vi "Find Mic Snippet.vi"() -> (0 "Mic B Device":dbl, 1 "Mic A Device":dbl, 2 "Number of Output Devices":i32, 3 "Number of Input Devices":i32, 4 "Speaker Device":dbl, 5 "Compensation factor":dbl, 6 "Faulty Mic":bool, 10 "Speaker Not Found":bool=TRUE)   [LabVIEW 2018]
uses:
  <vilib>/sound2/lvsound2.llb/Sound Data Format.ctl
  <vilib>/sound2/lvsound2.llb/Sampling Mode.ctl
  <vilib>/sound2/lvsound2.llb/Sound Output Set Volume (Single).vi
  <vilib>/sound2/lvsound2.llb/Sound Output Write (DBL Single).vi
  <vilib>/sound2/lvsound2.llb/Sound Input Read (DBL).vi
  <vilib>/addons/Sound and Vibration/svt_Level/SVT Sound Level (N Ch).vi
  <vilib>/measure/NI_MABase.lvlib
  <vilib>/addons/Sound and Vibration/svt_Level/SoundVib_SoundLevel.lvlib
panel:
  out "Filtered Signal 2":dynamicdata(graph) caption="Filtered Signal"
  out "Filtered Signal":dynamicdata(graph)
  out "db B":dbl
  out "db A":dbl
  out "Speaker Device 2":dbl
  out "equalized":dbl
  out "db Difference":dbl
  out "mv 2":dbl
  out "mv":dbl
  out "Number of Input Devices 2":i32
  in  "Boolean":bool
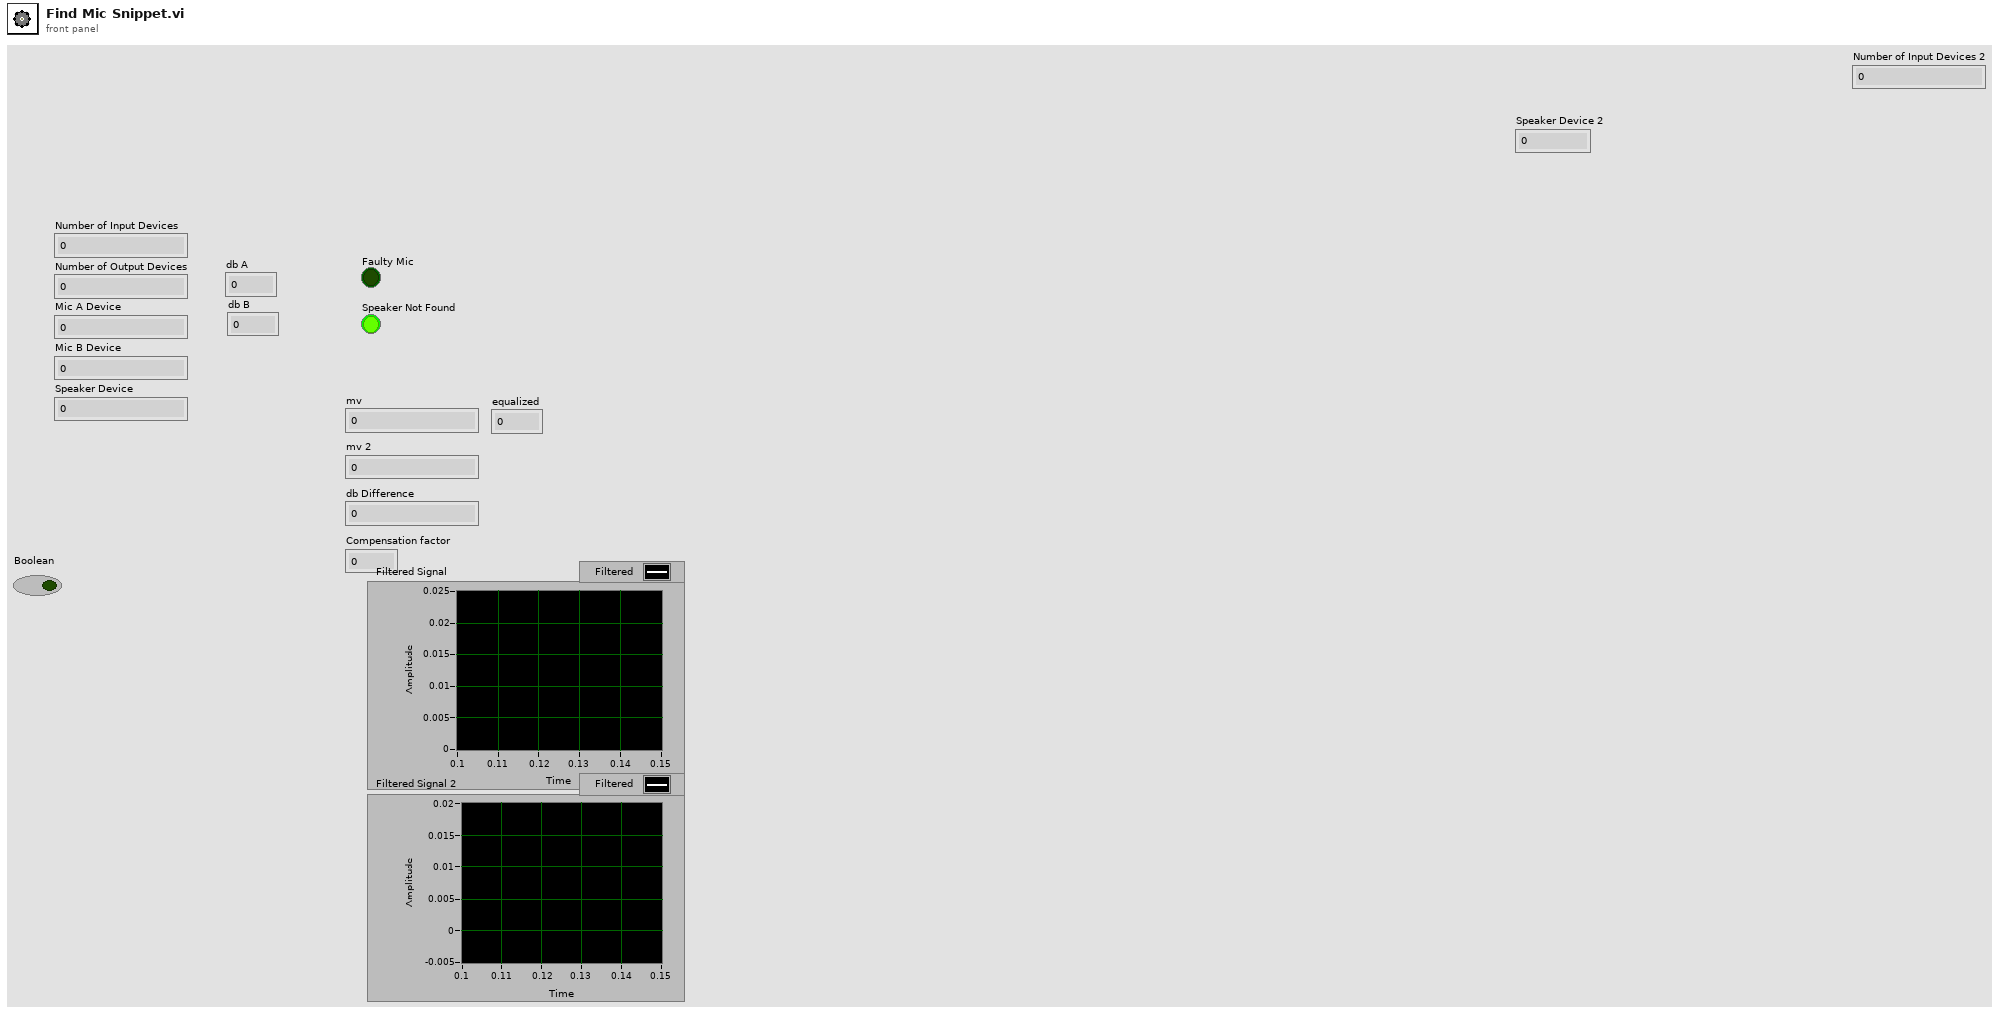
[diagram p1: front panel]
types:
  T1 = typedef "Sound Data Format.ctl" = cluster{"sample rate (S/s)":dbl, "number of channels":i32, "bits per sample":i32}
  T2 = cluster{"Leq":bool, "Running Leq":bool, "Exponential":bool, "Peak":bool}
  T3 = typedef "Sampling Mode.ctl" = i32
  T4 = typedef "Sound Output Task ID.ctl" = u32
  T5 = typedef "Sound Input Task ID.ctl" = u32
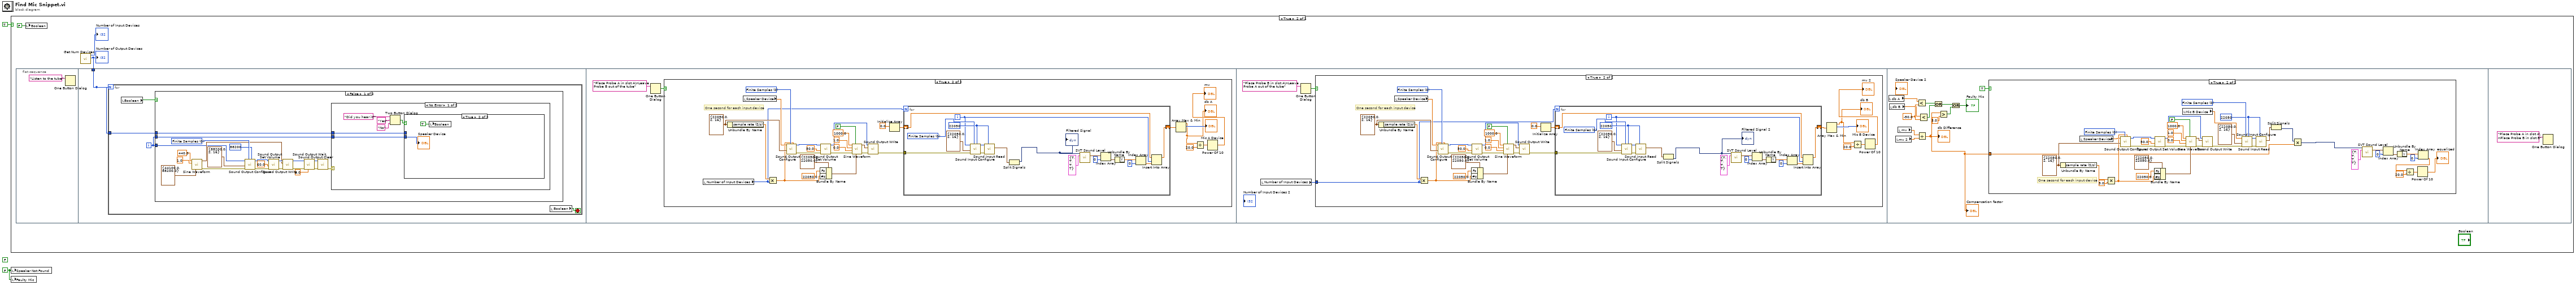
[diagram p0: block diagram]
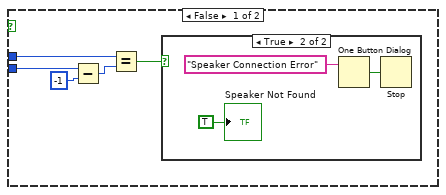
[diagram p3: hidden frame]
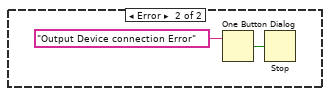
[diagram p5: hidden frame]
diagram:
  (unwired) FALSE
  w2 = FALSE
  n1 = case shown="True" TRUE {
    frame False {
    }
    frame True {
      n2 = flat-sequence {
        tunnel: w4 -> [w7]
        frame #0 {
          n3 = One Button Dialog(message="Listen to the tube") -> ()  [unwired: 1 in, 1 out]
        }
        frame #1 {
          n4 = for {
            N: w7 -> [_]
            tunnel: w7 -> [w8]
            i -> [w9]
            stop <- w11 stop-if-true
            n5 = local read "Boolean"() -> (w10:bool)
            n6 = case shown="False" w10 {
              tunnel: w9 -> [w14 _]
              tunnel: w9 -> [w13 _]
              tunnel: w8 -> [w12 _]
              frame False {
                w28 = T3 0 items=["Finite Samples", "Continuous Samples"] ("sample mode")
                n7 = call <vilib>:"Sine Waveform.vi"("sampling info"=cluster{"Fs":dbl, "#s":dbl} {"Fs"=44100.0, "#s"=88200.0}, "amplitude"=1.0, "frequency"=440.0) -> ("error out"=w31:errorcluster, "signal out"=w21:waveform(dbl))  [unwired: 7 in]
                n8 = call <vilib>:"Sound Output Configure.vi"("number of samples/ch"=88200, "sample mode"=w28, "error in (no error)"=w31, "sound format"=T1 {"sample rate (S/s)"=88200.0, "number of channels"=2, "bits per sample"=16}, "device ID"=w13) -> ("error out"=w26:errorcluster, "task ID"=w25:T4)  [unwired: 5 in]
                n9 = call-poly <vilib>:"Sound Output Set Volume.vi"("error in (no error)"=w26, "volume"=60.0, "task ID"=w25) -> ("error out"=w23:errorcluster, "task ID out"=w22:T4)  [unwired: 7 in]
                n10 = call-poly <vilib>:"Sound Output Write.vi"("error in (no error)"=w23, "data"=w21, "task ID"=w22) -> ("error out"=w20:errorcluster, "task ID out"=w19:T4)  [unwired: 7 in]
                n11 = call <vilib>:"Sound Output Wait.vi"("timeout (sec)"=2.0, "error in (no error)"=w20, "task ID"=w19) -> ("error out"=w17:errorcluster, "task ID out"=w16:T4)  [unwired: 7 in]
                n12 = call <vilib>:"Sound Output Clear.vi"("error in (no error)"=w17, "task ID"=w16) -> ("error out"=w15:errorcluster)  [unwired: 9 in]
                n13 = case shown="No Error" w15 {
                  tunnel: w14 -> [w35 _]
                  tunnel: w12 -> [w34 _]
                  frame No Error {
                    n14 = Two Button Dialog(message="Did you hear it?", 1:"No" ("F button name (\"Cancel\")"), 2:"Yes" ("T button name (\"OK\")")) -> (T button?=w36:bool)
                    n15 = case shown="True" w36 {
                      tunnel: w35 -> [w42 w48]
                      tunnel: w34 -> [w43 _]
                      frame False {
                        n16 = Subtract(x=w42, y=-1) -> (x-y=w40:i32)
                        n17 = Equal?(x=w43, y=w40) -> (x = y?=w44:bool)
                        n18 = case shown="True" w44 {
                          frame False {
                          }
                          frame True {
                            n19 = One Button Dialog(message="Speaker Connection Error") -> (true=w46:bool)  [unwired: 1 in]
                            n20 = Stop(stop? (T)=w46) -> ()
                            "Speaker Not Found" <- TRUE
                          }
                        }
                      }
                      frame True {
                        n21 = local write "Boolean"(TRUE ("Boolean")) -> ()
                        "Speaker Device" <- w48
                      }
                    }
                  }
                  frame Error {
                    n22 = One Button Dialog(message="Output Device connection Error") -> (true=w50:bool)  [unwired: 1 in]
                    n23 = Stop(stop? (T)=w50) -> ()
                  }
                }
              }
              frame True {
              }
            }
            n24 = local read "Boolean"() -> (w11:bool)
          }
        }
        frame #2 {
          n25 = One Button Dialog(message="Place Probe A in slot A\nLeave Probe B out of the tube") -> (true=w52:bool)  [unwired: 1 in]
          n26 = case shown="True" w52 {
            frame False {
            }
            frame True {
              w82 = T3 0 items=["Finite Samples", "Continuous Samples"] ("sample mode")
              w69 = T1 {"sample rate (S/s)"=22050.0, "number of channels"=2, "bits per sample"=16} ("sound format")
              # "One second for each input device"
              n27 = local read "Number of Input Devices"() -> (w63:i32)
              n28 = Unbundle By Name(w69) -> ("sample rate (S/s)"=w68:dbl)
              n29 = local read "Speaker Device"() -> (w79:dbl)
              n30 = Multiply(x=w68, y=w63) -> (x*y=w66:dbl)
              n31 = call <vilib>:"Sound Output Configure.vi"("number of samples/ch"=w66, "sample mode"=w82, "sound format"=w69, "device ID"=w79) -> ("error out"=w80:errorcluster, "task ID"=w81:T4)  [unwired: 6 in]
              n32 = Bundle By Name(cluster=cluster{"Fs":dbl, "#s":dbl} {"Fs"=22050.0, "#s"=22050.0} ("sampling info"), "Fs"=22050.0, "#s"=w66) -> (w64:cluster{"Fs":dbl, "#s":dbl})
              n33 = call-poly <vilib>:"Sound Output Set Volume.vi"("error in (no error)"=w80, "volume"=50.0, "task ID"=w81) -> ("error out"=w74:errorcluster, "task ID out"=w78:T4)  [unwired: 7 in]
              n34 = call <vilib>:"Sine Waveform.vi"("sampling info"=w64, "reset signal"=FALSE, "error in (no error)"=w74, "phase"=0.0, "amplitude"=1.0, "frequency"=1000.0) -> ("error out"=w73:errorcluster, "signal out"=w71:waveform(dbl))  [unwired: 4 in]
              n35 = call-poly <vilib>:"Sound Output Write.vi"("error in (no error)"=w73, "data"=w71, "task ID"=w78) -> ("error out"=w60:errorcluster)  [unwired: 7 in, 1 out]
              n36 = Initialize Array(0.0 ("element")) -> (w61:dbl[])  [unwired: 1 in]
              n37 = for {
                N: w63 -> [_]
                shift-right: [w88] -> w59
                shift-left: w61 -> [w89]
                tunnel: w60 -> [w85]
                i -> [w86]
                w96 = 22050 ("number of samples/ch")
                w99 = T3 0 items=["Finite Samples", "Continuous Samples"] ("sample mode")
                n38 = call <vilib>:"Sound Input Configure.vi"("number of samples/ch"=w96, "sample mode"=w99, "error in (no error)"=w85, "sound format"=T1 {"sample rate (S/s)"=22050.0, "number of channels"=2, "bits per sample"=16}, "device ID"=w86) -> ("error out"=w98:errorcluster, "task ID"=w97:T5)  [unwired: 5 in]
                n39 = call-poly <vilib>:"Sound Input Read.vi"("number of samples/ch"=w96, "error in (no error)"=w98, "task ID"=w97) -> ("data"=w84:waveform(dbl)[])  [unwired: 6 in, 2 out]
                n40 = Split Signals(w84) -> (w83:dynamicdata)  [unwired: 2 in, 1 out]
                "Filtered Signal" <- w83
                n41 = call-poly <vilib>:"SVT Sound Level.vi"("scaled signals [EU]"=w83, "measurement selection"=T2 {"Leq"=TRUE, "Running Leq"=TRUE, "Exponential"=TRUE, "Peak"=TRUE}) -> ("running Leq sound levels [dB EU]"=w94:waveform(dbl)[])  [unwired: 8 in, 5 out]
                n42 = Index Array(array=w94, index=0) -> (element=w92:waveform(dbl))
                n43 = Unbundle By Name(w92) -> ("Y"=w90:dbl[])
                n44 = Index Array(array=w90, index=0) -> (element=w87:dbl)
                n45 = Insert Into Array(array=w89, index=w86, new element=w87) -> (w88:dbl[])
              }
              n46 = Array Max & Min(array=w59) -> (max value=w54:dbl, max index (indices)=→"Mic A Device":i32)  [unwired: 2 out]
              "db A" <- w54
              n47 = Divide(x=w54, y=20.0) -> (x/y=w57:dbl)
              n48 = Power Of 10(x=w57) -> (10^x=→"mv":dbl)
            }
          }
        }
        frame #3 {
          n49 = local read "Number of Input Devices"() -> (w103:i32)
          n50 = One Button Dialog(message="Place Probe B in slot A\nLeave Probe A out of the tube") -> (true=w101:bool)  [unwired: 1 in]
          n51 = case shown="True" w101 {
            tunnel: w103 -> [_ w109]
            frame False {
            }
            frame True {
              w132 = T3 0 items=["Finite Samples", "Continuous Samples"] ("sample mode")
              w119 = T1 {"sample rate (S/s)"=22050.0, "number of channels"=2, "bits per sample"=16} ("sound format")
              # "One second for each input device"
              n52 = Unbundle By Name(w119) -> ("sample rate (S/s)"=w118:dbl)
              n53 = local read "Speaker Device"() -> (w129:dbl)
              n54 = Multiply(x=w118, y=w109) -> (x*y=w116:dbl)
              n55 = call <vilib>:"Sound Output Configure.vi"("number of samples/ch"=w116, "sample mode"=w132, "sound format"=w119, "device ID"=w129) -> ("error out"=w130:errorcluster, "task ID"=w131:T4)  [unwired: 6 in]
              n56 = Bundle By Name(cluster=cluster{"Fs":dbl, "#s":dbl} {"Fs"=22050.0, "#s"=22050.0} ("sampling info"), "Fs"=22050.0, "#s"=w116) -> (w114:cluster{"Fs":dbl, "#s":dbl})
              n57 = call-poly <vilib>:"Sound Output Set Volume.vi"("error in (no error)"=w130, "volume"=50.0, "task ID"=w131) -> ("error out"=w124:errorcluster, "task ID out"=w128:T4)  [unwired: 7 in]
              n58 = call <vilib>:"Sine Waveform.vi"("sampling info"=w114, "reset signal"=FALSE, "error in (no error)"=w124, "phase"=0.0, "amplitude"=1.0, "frequency"=1000.0) -> ("error out"=w123:errorcluster, "signal out"=w121:waveform(dbl))  [unwired: 4 in]
              n59 = call-poly <vilib>:"Sound Output Write.vi"("error in (no error)"=w123, "data"=w121, "task ID"=w128) -> ("error out"=w111:errorcluster)  [unwired: 7 in, 1 out]
              n60 = Initialize Array(0.0 ("element")) -> (w112:dbl[])  [unwired: 1 in]
              n61 = for {
                N: w109 -> [_]
                shift-right: [w138] -> w110
                shift-left: w112 -> [w139]
                tunnel: w111 -> [w135]
                i -> [w136]
                w146 = 22050 ("number of samples/ch")
                w149 = T3 0 items=["Finite Samples", "Continuous Samples"] ("sample mode")
                n62 = call <vilib>:"Sound Input Configure.vi"("number of samples/ch"=w146, "sample mode"=w149, "error in (no error)"=w135, "sound format"=T1 {"sample rate (S/s)"=22050.0, "number of channels"=2, "bits per sample"=16}, "device ID"=w136) -> ("error out"=w148:errorcluster, "task ID"=w147:T5)  [unwired: 5 in]
                n63 = call-poly <vilib>:"Sound Input Read.vi"("number of samples/ch"=w146, "error in (no error)"=w148, "task ID"=w147) -> ("data"=w134:waveform(dbl)[])  [unwired: 6 in, 2 out]
                n64 = Split Signals(w134) -> (w133:dynamicdata)  [unwired: 2 in, 1 out]
                "Filtered Signal 2" <- w133
                n65 = call-poly <vilib>:"SVT Sound Level.vi"("scaled signals [EU]"=w133, "measurement selection"=T2 {"Leq"=TRUE, "Running Leq"=TRUE, "Exponential"=TRUE, "Peak"=TRUE}) -> ("running Leq sound levels [dB EU]"=w144:waveform(dbl)[])  [unwired: 8 in, 5 out]
                n66 = Index Array(array=w144, index=0) -> (element=w142:waveform(dbl))
                n67 = Unbundle By Name(w142) -> ("Y"=w140:dbl[])
                n68 = Index Array(array=w140, index=0) -> (element=w137:dbl)
                n69 = Insert Into Array(array=w139, index=w136, new element=w137) -> (w138:dbl[])
              }
              n70 = Array Max & Min(array=w110) -> (max value=w104:dbl, max index (indices)=→"Mic B Device":i32)  [unwired: 2 out]
              "db B" <- w104
              n71 = Divide(x=w104, y=20.0) -> (x/y=w107:dbl)
              n72 = Power Of 10(x=w107) -> (10^x=→"mv 2":dbl)
            }
          }
        }
        frame #4 {
          w162 = -50.0 ("y")
          n73 = local read "db A"() -> (w155:dbl)
          n74 = local read "db B"() -> (w154:dbl)
          n75 = local read "mv 2"() -> (w152:dbl)
          n76 = local read "mv"() -> (w153:dbl)
          n77 = Less?(x=w155, y=w162) -> (x < y?=w161:bool)
          n78 = Divide(x=w153, y=w152) -> (x/y=w151:dbl)
          "db Difference" <- w151
          "Compensation factor" <- w151
          n79 = Less?(x=w154, y=w162) -> (x < y?=w160:bool)
          n80 = Or(x=w161, y=w160) -> (x .or. y?=w159:bool)
          n81 = Greater?(x=w151, y=3.0) -> (0:w157:bool)
          n82 = Or(x=w159, y=w157) -> (x .or. y?=→"Faulty Mic":bool)
          n83 = case shown="True" TRUE {
            tunnel: w151 -> [_ w171]
            frame False {
            }
            frame True {
              w180 = 22050 ("number of samples/ch")
              w183 = T3 0 items=["Finite Samples", "Continuous Samples"] ("sample mode")
              w204 = T3 0 items=["Finite Samples", "Continuous Samples"] ("sample mode")
              w191 = T1 {"sample rate (S/s)"=22050.0, "number of channels"=2, "bits per sample"=16} ("sound format")
              # "One second for each input device"
              n84 = Unbundle By Name(w191) -> ("sample rate (S/s)"=w190:dbl)
              n85 = local read "Speaker Device"() -> (w201:dbl)
              n86 = Multiply(x=w190, y=3.0) -> (x*y=w188:dbl)
              n87 = call <vilib>:"Sound Output Configure.vi"("number of samples/ch"=w188, "sample mode"=w204, "sound format"=w191, "device ID"=w201) -> ("error out"=w202:errorcluster, "task ID"=w203:T4)  [unwired: 6 in]
              n88 = Bundle By Name(cluster=cluster{"Fs":dbl, "#s":dbl} {"Fs"=22050.0, "#s"=22050.0} ("sampling info"), "Fs"=22050.0, "#s"=w188) -> (w186:cluster{"Fs":dbl, "#s":dbl})
              n89 = call-poly <vilib>:"Sound Output Set Volume.vi"("error in (no error)"=w202, "volume"=50.0, "task ID"=w203) -> ("error out"=w196:errorcluster, "task ID out"=w200:T4)  [unwired: 7 in]
              n90 = local read "Mic B Device"() -> (w173:dbl)
              n91 = call <vilib>:"Sine Waveform.vi"("sampling info"=w186, "reset signal"=FALSE, "error in (no error)"=w196, "phase"=0.0, "amplitude"=1.0, "frequency"=1000.0) -> ("error out"=w195:errorcluster, "signal out"=w193:waveform(dbl))  [unwired: 4 in]
              n92 = call-poly <vilib>:"Sound Output Write.vi"("error in (no error)"=w195, "data"=w193, "task ID"=w200) -> ("error out"=w185:errorcluster)  [unwired: 7 in, 1 out]
              n93 = call <vilib>:"Sound Input Configure.vi"("number of samples/ch"=w180, "sample mode"=w183, "error in (no error)"=w185, "sound format"=T1 {"sample rate (S/s)"=22050.0, "number of channels"=2, "bits per sample"=16}, "device ID"=w173) -> ("error out"=w182:errorcluster, "task ID"=w181:T5)  [unwired: 5 in]
              n94 = call-poly <vilib>:"Sound Input Read.vi"("number of samples/ch"=w180, "error in (no error)"=w182, "task ID"=w181) -> ("data"=w166:waveform(dbl)[])  [unwired: 6 in, 2 out]
              n95 = Split Signals(w166) -> (w165:dynamicdata)  [unwired: 2 in, 1 out]
              n96 = Multiply(x=w165, y=w171) -> (x*y=w164:dynamicdata)
              n97 = call-poly <vilib>:"SVT Sound Level.vi"("scaled signals [EU]"=w164, "measurement selection"=T2 {"Leq"=TRUE, "Running Leq"=TRUE, "Exponential"=TRUE, "Peak"=TRUE}) -> ("running Leq sound levels [dB EU]"=w178:waveform(dbl)[])  [unwired: 8 in, 5 out]
              n98 = Index Array(array=w178, index=0) -> (element=w176:waveform(dbl))
              n99 = Unbundle By Name(w176) -> ("Y"=w174:dbl[])
              n100 = Index Array(array=w174, index=0) -> (element=w168:dbl)
              n101 = Divide(x=w168, y=20.0) -> (x/y=w170:dbl)
              n102 = Power Of 10(x=w170) -> (10^x=→"equalized":dbl)
            }
          }
        }
        frame #5 {
          n103 = One Button Dialog(message="Place Probe A in slot A\nPlace Probe B in slot B") -> ()  [unwired: 1 in, 1 out]
        }
      }
      n104 = local write "Boolean"(FALSE ("Boolean")) -> ()
      n105 = call <vilib>:"Get Num Devices.vi"() -> ("Number of Output Devices"=w4:i32, "Number of Input Devices"=→"Number of Input Devices":i32)  [unwired: 9 in, 1 out]
      "Number of Output Devices" <- w4
    }
  }
  n106 = local write "Speaker Not Found"(w2) -> ()
  n107 = local write "Faulty Mic"(w2) -> ()
